vi "DVR Create.vi"(8 "error in (no error)":errorcluster, 11 "UI_Top_Customer in":refnum<class "UI_Top_Customer.lvclass">) -> (0 "error out":errorcluster, 3 "UI_Top_Customer out":refnum<class "UI_Top_Customer.lvclass">)   [LabVIEW 2021, in "UI_Top_Customer.lvclass"]
uses:
  UI_Top_Customer.lvclass
  Pane MouseDown.ctl
  <vilib>/event_ctls.llb/lveventtype.ctl
  <vilib>/Utility/miscctls.llb/LVPoint32TypeDef.ctl
  UI_Top_Customer.lvclass/UI_Top_Customer.ctl
  Z:/UTP_2023/Source_OPCUA_Server/UI_Left_Right/UI_Left_Right.lvclass
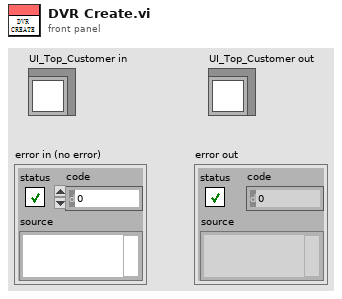
[diagram p1: front panel]
types:
  T1 = typedef "UI_Top_Customer.lvclass/Pane MouseDown.ctl" = cluster{"Type":T2, "Coords":T3, "Mods":cluster{"Double Click":bool, "Menu Key":bool}, "Pane: MouseDown":bool}
  T2 = typedef "lveventtype.ctl" = enum32{"Null", "Timeout", "Annotation Menu Selection", "Annotation Menu Selection?", "App Instance Close", "App Instance Close?", "Autoscale Range Change", "Bookmark Info Change", "Cell Edit", "Cell Edit?", "Cursor Grab", "Cursor Grab?", "Cursor Menu Selection", "Cursor Menu Selection?", "Cursor Move", "Cursor Release", "Data Change", "Direction Change", "Display State Change", "Drag Ended", "Drag Enter", "Drag Leave", "Drag Over", "Drag Source Update", "Drag Starting", "Drag Starting?", "Drop", "Exec State Change", "Key Down", "Key Down?", "Key Repeat", "Key Repeat?", "Key Up", "Listbox Double Click", "Menu Activation?", "Menu Selection (App)", "Menu Selection? (App)", "Menu Selection (User)", "Mouse Down", "Mouse Down?", "Mouse Enter", "Mouse Leave", "Mouse Move", "Mouse Up", "Mouse Wheel", "NI Security User Change (App)", "Pane Size", "Panel Close", "Panel Close?", "Panel Resize", "Plot Attribute Change", "Scale Range Change", "Shortcut Menu Activation?", "Shortcut Menu Selection (App)", "Shortcut Menu Selection? (App)", "Shortcut Menu Selection (User)", "Tree Double Click", "Tree Drag", "Tree Drag?", "Tree Drop", "Tree Drop?", "Tree Item Close", "Tree Item Close?", "Tree Item Open", "Tree Item Open?", "User Event", "Value Change"}
  T3 = typedef "UI_LeftRight.lvlib/UI_Left_Right.lvclass/LVPoint32TypeDef.ctl" = cluster{"Horizontal":i32, "Vertical":i32}
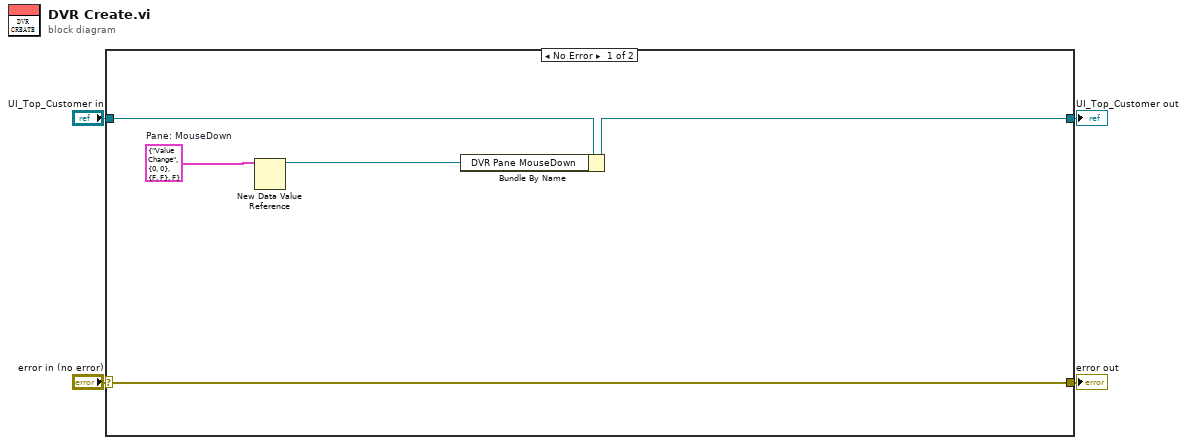
[diagram p0: block diagram]
diagram:
  n1 = case shown="No Error" "error in (no error)" {
    selector: "error in (no error)" -> [w8 w11]
    tunnel: [w8 w11] -> w3
    tunnel: [w7 w10] -> w1
    tunnel: "UI_Top_Customer in" -> [w9 w10]
    frame No Error {
      w6 = T1 {"Type"=enum."Value Change", "Coords"={"Horizontal"=0, "Vertical"=0}, "Mods"={"Double Click"=FALSE, "Menu Key"=FALSE}, "Pane: MouseDown"=FALSE}  # Pane: MouseDown
      n2 = New Data Value Reference(data value=w6) -> (data value reference=w5:refnum<data-value>)  [unwired: 1 in, 1 out]
      n3 = Bundle By Name(cluster=w9, "DVR Pane MouseDown"=w5) -> (w7:refnum<class "UI_Top_Customer.lvclass">)
    }
    frame Error {
    }
  }
  "error out" <- w3
  "UI_Top_Customer out" <- w1
